vi "MRC Systemcore Get Team Number.vi"(8 "error in (no error)":errorcluster) -> (0 "error out":errorcluster, 3 "team":T1)   [LabVIEW 2026, in "MrcLib.lvlib"]
doc: "MRC_Status MRC_CALLCONV MRC_Systemcore_GetBatteryVoltage(float* voltage);"
uses:
  MrcLib.lvlib
  Types/MRC String.ctl
  MrcLib.dll
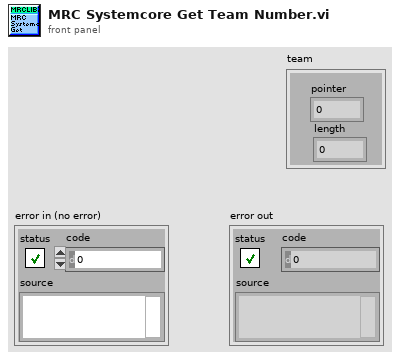
[diagram p1: front panel]
types:
  T1 = typedef "MRC String.ctl" = cluster{"pointer":u64, "length":u64}
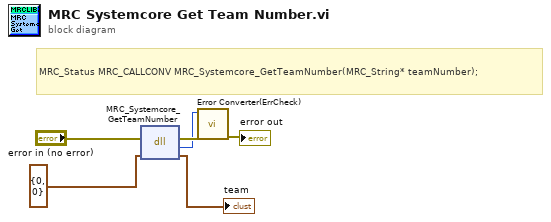
[diagram p0: block diagram]
diagram:
  # "MRC_Status MRC_CALLCONV MRC_Systemcore_GetTeamNumber(MRC_String* teamNumber);"
  n1 = dll-call lib="MrcLib.*" fn="MRC_Systemcore_GetTeamNumber"(error in="error in (no error)", "string"=T1 {"pointer"=0, "length"=0} ("message")) -> (error out=w5:errorcluster, "return type"=w3:i32, "string"=→"team":T1)  [unwired: 2 in, 1 out]
  n2 = call "Error Converter(ErrCheck).vi"("error in (no error)"=w5, "status"=w3) -> ("error out"=→"error out":errorcluster)  [unwired: 9 in]
